vi "Target Select with keyboard.vi"(0 "High":bool, 5 "Right":bool, 7 "Left":bool, 9 "Low":bool, 11 "Pyramid":bool) -> (4 "1":bool, 6 "2":bool, 8 "3":bool, 10 "4":bool, 14 "Selected Goal":i32=1, 15 "5":bool)   [LabVIEW 2012]
uses:
  Keys Pressed Global.vi
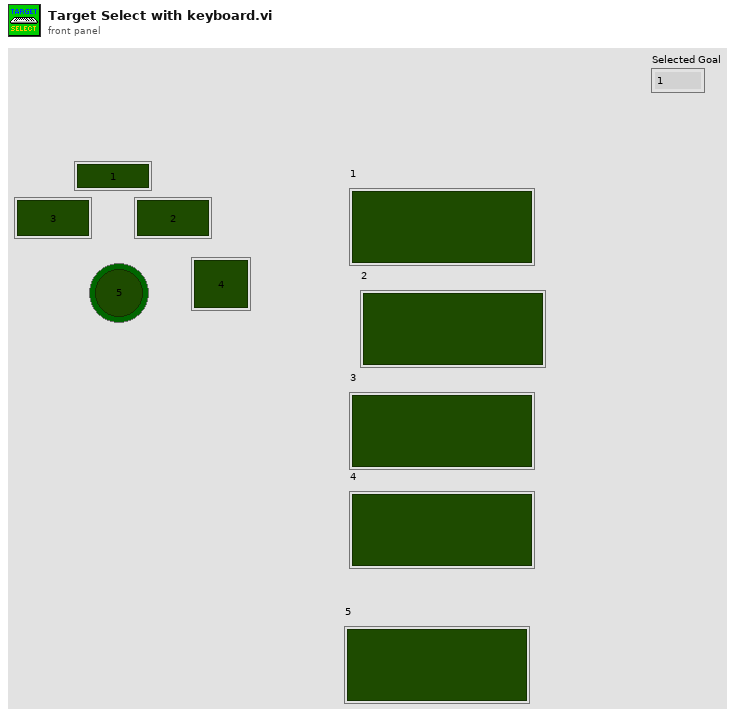
[diagram p1: front panel]
types:
  T1 = enum16{"0", "1", "2", "3", "4", "5", "6", "7", "8", "9", "A", "B", "C", "D", "E", "F", "G", "H", "I", "J", "K", "L", "M", "N", "O", "P", "Q", "R", "S", "T", "U", "V", "W", "X", "Y", "Z", "F1", "F2", "F3", "F4", "F5", "F6", "F7", "F8", "F9", "F10", "F11", "F12", "F13", "F14", "F15", "ADD", "BACK", "BACKSLASH", "CAPITAL", "COMMA", "DECIMAL", "DELETE", "DIVIDE", "DOWN", "END", "EQUALS", "ESCAPE", "GRAVE (`)", "HOME", "INSERT", "LBRACKET", "LCONTROL", "LEFT", "L ALT", "LSHIFT", "LWIN", "MINUS", "MULTIPLY", "NEXT", "NUMLOCK", "NUMPAD_0", "NUMPAD_1", "NUMPAD_2", "NUMPAD_3", "NUMPAD_4", "NUMPAD_5", "NUMPAD_6", "NUMPAD_7", "NUMPAD_8", "NUMPAD_9", "PAUSE", "PERIOD", "PRIOR (PG UP)", "RBRACKET", "RCONTROL", "RETURN", "RIGHT", "R ALT", "RSHIFT", "RWIN", "SCROLL", "SEMICOLON", "SLASH", "SPACE", "SUBTRACT", "TAB", "UP", "ENTER (num pad)", "' (quote)"}
  T2 = enum16{"0", "1", "2", "3", "4", "5", "6", "7", "8", "9", "A", "B", "C", "D", "E", "F", "G", "H", "I", "J", "K", "L", "M", "N", "O", "P", "Q", "R", "S", "T", "U", "V", "W", "X", "Y", "Z", "F1", "F2", "F3", "F4", "F5", "F6", "F7", "F8", "F9", "F10", "F11", "F12", "F13", "F14", "F15", "ADD", "BACK", "BACKSLASH", "CAPITAL", "COMMA", "DECIMAL", "DELETE", "DIVIDE", "DOWN", "END", "EQUALS", "ESCAPE", "GRAVE (`)", "HOME", "INSERT", "LBRACKET", "LCONTROL", "LEFT", "L ALT", "LSHIFT", "LWIN", "MINUS", "MULTIPLY", "NEXT", "NUMLOCK", "NUMPAD_0", "NUMPAD_1", "NUMPAD_2", "NUMPAD_3", "NUMPAD_4", "NUMPAD_5", "NUMPAD_6", "NUMPAD_7", "NUMPAD_8", "NUMPAD_9", "PAUSE", "PERIOD", "PRIOR (PG UP)", "RBRACKET", "RCONTROL", "RETURN", "RIGHT", "R ALT", "RSHIFT", "RWIN", "SCROLL", "SEMICOLON", "SLASH", "SPACE", "SUBTRACT", "TAB", "UP", "ENTER (num pad)", "' (quote)"}[]
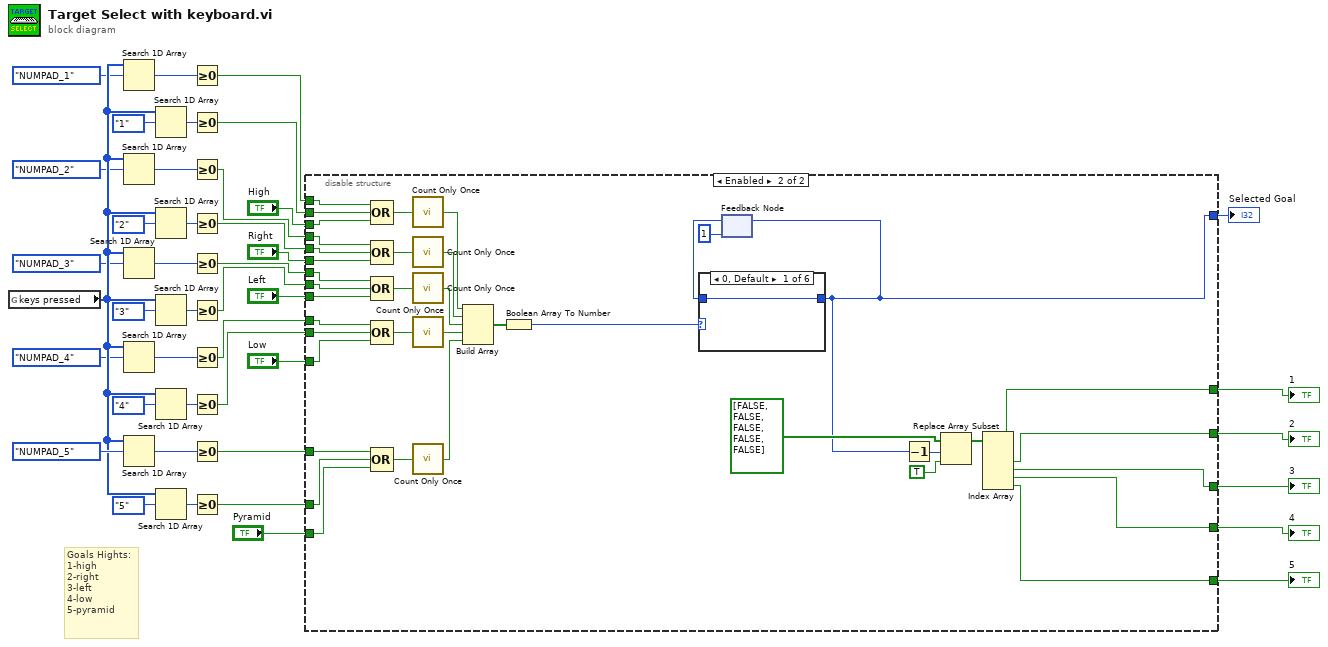
[diagram p0: block diagram]
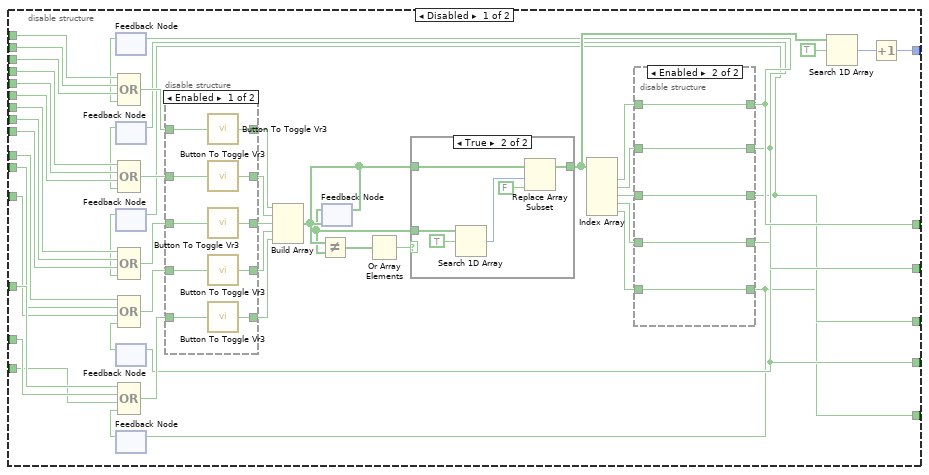
[diagram p2: hidden frame]
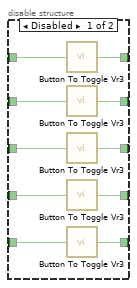
[diagram p4: hidden frame]
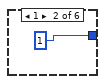
[diagram p6: hidden frame]
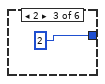
[diagram p7: hidden frame]
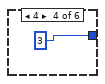
[diagram p8: hidden frame]
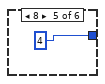
[diagram p9: hidden frame]
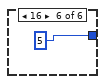
[diagram p10: hidden frame]
diagram:
  # "Goals Hights:\n1-high\n2-right\n3-left\n4-low\n5-pyramid"
  n1 = global read "Keys Pressed Global.vi" "keys pressed"() -> (w36:T2)
  n2 = Search 1D Array(1D array=w36, element=T1."NUMPAD_1" ("keys pressed[0]")) -> (index of element=w19:i32)  [unwired: 1 in]
  n3 = Search 1D Array(1D array=w36, element=T1."NUMPAD_2" ("keys pressed[0]")) -> (index of element=w26:i32)  [unwired: 1 in]
  n4 = Search 1D Array(1D array=w36, element=T1."NUMPAD_3" ("keys pressed[0]")) -> (index of element=w27:i32)  [unwired: 1 in]
  n5 = Search 1D Array(1D array=w36, element=T1."NUMPAD_4" ("keys pressed[0]")) -> (index of element=w34:i32)  [unwired: 1 in]
  n6 = Search 1D Array(1D array=w36, element=T1."NUMPAD_5" ("keys pressed[0]")) -> (index of element=w37:i32)  [unwired: 1 in]
  n7 = Search 1D Array(1D array=w36, element=T1."1" ("keys pressed[0]")) -> (index of element=w22:i32)  [unwired: 1 in]
  n8 = Search 1D Array(1D array=w36, element=T1."2" ("keys pressed[0]")) -> (index of element=w23:i32)  [unwired: 1 in]
  n9 = Search 1D Array(1D array=w36, element=T1."3" ("keys pressed[0]")) -> (index of element=w30:i32)  [unwired: 1 in]
  n10 = Search 1D Array(1D array=w36, element=T1."4" ("keys pressed[0]")) -> (index of element=w31:i32)  [unwired: 1 in]
  n11 = Search 1D Array(1D array=w36, element=T1."5" ("keys pressed[0]")) -> (index of element=w40:i32)  [unwired: 1 in]
  n12 = Greater Or Equal To 0?(x=w19) -> (x >= 0?=w18:bool)
  n13 = Greater Or Equal To 0?(x=w22) -> (x >= 0?=w17:bool)
  n14 = Greater Or Equal To 0?(x=w26) -> (x >= 0?=w15:bool)
  n15 = Greater Or Equal To 0?(x=w23) -> (x >= 0?=w14:bool)
  n16 = Greater Or Equal To 0?(x=w27) -> (x >= 0?=w12:bool)
  n17 = Greater Or Equal To 0?(x=w30) -> (x >= 0?=w11:bool)
  n18 = Greater Or Equal To 0?(x=w34) -> (x >= 0?=w10:bool)
  n19 = Greater Or Equal To 0?(x=w31) -> (x >= 0?=w9:bool)
  n20 = Greater Or Equal To 0?(x=w37) -> (x >= 0?=w41:bool)
  n21 = Greater Or Equal To 0?(x=w40) -> (x >= 0?=w42:bool)
  n22 = disable-structure shown="Enabled" {
    disable-tunnel: w42 -> [w90 w153]
    disable-tunnel: w41 -> [w89 w152]
    disable-tunnel: "Pyramid" -> [w88 w154]
    disable-tunnel: w18 -> [w87 w166]
    disable-tunnel: w17 -> [w86 w165]
    disable-tunnel: "High" -> [w85 w164]
    disable-tunnel: w15 -> [w84 w163]
    disable-tunnel: w14 -> [w83 w162]
    disable-tunnel: "Right" -> [w82 w161]
    disable-tunnel: w12 -> [w81 w160]
    disable-tunnel: w11 -> [w80 w159]
    disable-tunnel: w10 -> [w79 w157]
    disable-tunnel: w9 -> [w78 w156]
    disable-tunnel: "Left" -> [w77 w158]
    disable-tunnel: "Low" -> [w76 w155]
    disable-tunnel: [w49 w136] -> w6
    disable-tunnel: [w47 w132] -> w5
    disable-tunnel: [w46 w131] -> w4
    disable-tunnel: [w45 w130] -> w3
    disable-tunnel: [w44 w129] -> w2
    disable-tunnel: [w43 w128] -> w1
    frame Disabled {
      n23 = feedback #1() -> (w53:bool)  [unwired: 1 in]
      n24 = feedback #2() -> (w52:bool)  [unwired: 1 in]
      n25 = feedback #3() -> (w54:bool)  [unwired: 1 in]
      n26 = feedback #4() -> (w55:bool)  [unwired: 1 in]
      n27 = feedback #5() -> (w56:bool)  [unwired: 1 in]
      n28 = Compound Arithmetic op=OR(w87, w86, w85, w53) -> (w65:bool)
      n29 = Compound Arithmetic op=OR(w84, w83, w82, w52) -> (w64:bool)
      n30 = Compound Arithmetic op=OR(w81, w80, w77, w54) -> (w63:bool)
      n31 = Compound Arithmetic op=OR(w79, w78, w76, w55) -> (w62:bool)
      n32 = Compound Arithmetic op=OR(w89, w90, w88, w56) -> (w61:bool)
      n33 = disable-structure shown="Enabled" {
        disable-tunnel: w65 -> [w122 w127]
        disable-tunnel: w64 -> [w121 w126]
        disable-tunnel: w63 -> [w120 w125]
        disable-tunnel: w62 -> [w119 w124]
        disable-tunnel: w61 -> [w118 w123]
        disable-tunnel: [w117 w127] -> w72
        disable-tunnel: [w116 w126] -> w71
        disable-tunnel: [w115 w125] -> w75
        disable-tunnel: [w114 w124] -> w74
        disable-tunnel: [w113 w123] -> w73
        frame Enabled {
          n34 = call "Button To Toggle Vr3.vi"("InValue"=w122) -> ("Result"=w117:bool)
          n35 = call "Button To Toggle Vr3.vi"("InValue"=w121) -> ("Result"=w116:bool)
          n36 = call "Button To Toggle Vr3.vi"("InValue"=w120) -> ("Result"=w115:bool)
          n37 = call "Button To Toggle Vr3.vi"("InValue"=w119) -> ("Result"=w114:bool)
          n38 = call "Button To Toggle Vr3.vi"("InValue"=w118) -> ("Result"=w113:bool)
        }
        frame Disabled {
        }
      }
      n39 = Build Array(w72, w71, w75, w74, w73) -> (w58:bool[])
      n40 = feedback #6(w58) -> (w57:bool[])
      n41 = Not Equal?(x=w58, y=w57) -> (x != y?=w60:bool[])
      n42 = feedback-in #6(w58) -> ()
      n43 = Or Array Elements(Boolean array=w60) -> (logical OR=w59:bool)
      n44 = case shown="True" w59 {
        tunnel: w57 -> [_ w96]
        tunnel: w58 -> [w91 w95]
        tunnel: [w91 w92] -> w51
        frame False {
        }
        frame True {
          n45 = Search 1D Array(1D array=w96, element=TRUE) -> (index of element=w94:i32)  [unwired: 1 in]
          n46 = Replace Array Subset(array=w95, new element=FALSE ("new element/subarray"), index=w94) -> (w92:bool[])
        }
      }
      n47 = Index Array(array=w51) -> (element #1=w70:bool, element #2=w69:bool, element #3=w68:bool, element #4=w67:bool, element #5=w66:bool)  [unwired: 5 in]
      n48 = disable-structure shown="Enabled" {
        disable-tunnel: w70 -> [w107 w112]
        disable-tunnel: w69 -> [w106 w111]
        disable-tunnel: w68 -> [w105 w110]
        disable-tunnel: w67 -> [w104 w109]
        disable-tunnel: w66 -> [w103 w108]
        disable-tunnel: [w102 w112] -> w47
        disable-tunnel: [w101 w111] -> w46
        disable-tunnel: [w100 w110] -> w45
        disable-tunnel: [w99 w109] -> w44
        disable-tunnel: [w98 w108] -> w43
        frame Disabled {
          n49 = call "Button To Toggle Vr3.vi"("InValue"=w107) -> ("Result"=w102:bool)
          n50 = call "Button To Toggle Vr3.vi"("InValue"=w106) -> ("Result"=w101:bool)
          n51 = call "Button To Toggle Vr3.vi"("InValue"=w105) -> ("Result"=w100:bool)
          n52 = call "Button To Toggle Vr3.vi"("InValue"=w104) -> ("Result"=w99:bool)
          n53 = call "Button To Toggle Vr3.vi"("InValue"=w103) -> ("Result"=w98:bool)
        }
        frame Enabled {
        }
      }
      n54 = feedback-in #1(w47) -> ()
      n55 = feedback-in #2(w46) -> ()
      n56 = feedback-in #3(w45) -> ()
      n57 = feedback-in #4(w44) -> ()
      n58 = feedback-in #5(w43) -> ()
      n59 = Search 1D Array(1D array=w51, element=TRUE) -> (index of element=w50:i32)  [unwired: 1 in]
      n60 = Increment(x=w50) -> (x+1=w49:i32)
    }
    frame Enabled {
      n61 = Compound Arithmetic op=OR(w166, w165, w164) -> (w147:bool)
      n62 = Compound Arithmetic op=OR(w163, w162, w161) -> (w146:bool)
      n63 = Compound Arithmetic op=OR(w160, w159, w158) -> (w144:bool)
      n64 = Compound Arithmetic op=OR(w157, w156, w155) -> (w142:bool)
      n65 = Compound Arithmetic op=OR(w152, w153, w154) -> (w140:bool)
      n66 = call "Count Only Once.vi"("InValue"=w147) -> ("Result"=w148:bool)
      n67 = call "Count Only Once.vi"("InValue"=w146) -> ("Result"=w145:bool)
      n68 = call "Count Only Once.vi"("InValue"=w144) -> ("Result"=w143:bool)
      n69 = call "Count Only Once.vi"("InValue"=w142) -> ("Result"=w141:bool)
      n70 = call "Count Only Once.vi"("InValue"=w140) -> ("Result"=w139:bool)
      n71 = Build Array(w148, w145, w143, w141, w139) -> (w151:bool[])
      n72 = Boolean Array To Number(Boolean array=w151) -> (number=w150:u32)
      n73 = feedback #7(1 ("Selected Goal")) -> (w149:i32)
      n74 = case shown="0, Default" w150 {
        tunnel: [w167 1 ("Selected Goal") 2 ("Selected Goal") 3 ("Selected Goal") 4 ("Selected Goal") 5 ("Selected Goal")] -> w136
        tunnel: w149 -> [w167 _ _ _ _ _]
        frame 0, Default {
        }
        frame 1 {
        }
        frame 2 {
        }
        frame 4 {
        }
        frame 8 {
        }
        frame 16 {
        }
      }
      n75 = feedback-in #7(w136) -> ()
      n76 = Decrement(x=w136) -> (x-1=w135:i32)
      n77 = Replace Array Subset(array=bool[] [FALSE, FALSE, FALSE, FALSE, FALSE], new element=TRUE ("new element/subarray"), index=w135) -> (w133:bool[])
      n78 = Index Array(array=w133) -> (element #1=w132:bool, element #2=w131:bool, element #3=w130:bool, element #4=w129:bool, element #5=w128:bool)  [unwired: 5 in]
    }
  }
  "Selected Goal" <- w6
  "5" <- w1
  "1" <- w5
  "2" <- w4
  "3" <- w3
  "4" <- w2
